vi "RT_MATH_IIR_Filt.vi"(4 "Data In":sgl, 5 "Filter Response (rad/s)":sgl, 6 "Iteration Time Delta(s)":sgl, 7 "Last Data Out":sgl) -> (2 "RC":sgl, 3 "Data Out":sgl)   [LabVIEW 2024]
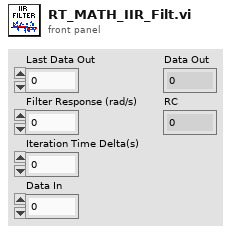
[diagram p1: front panel]
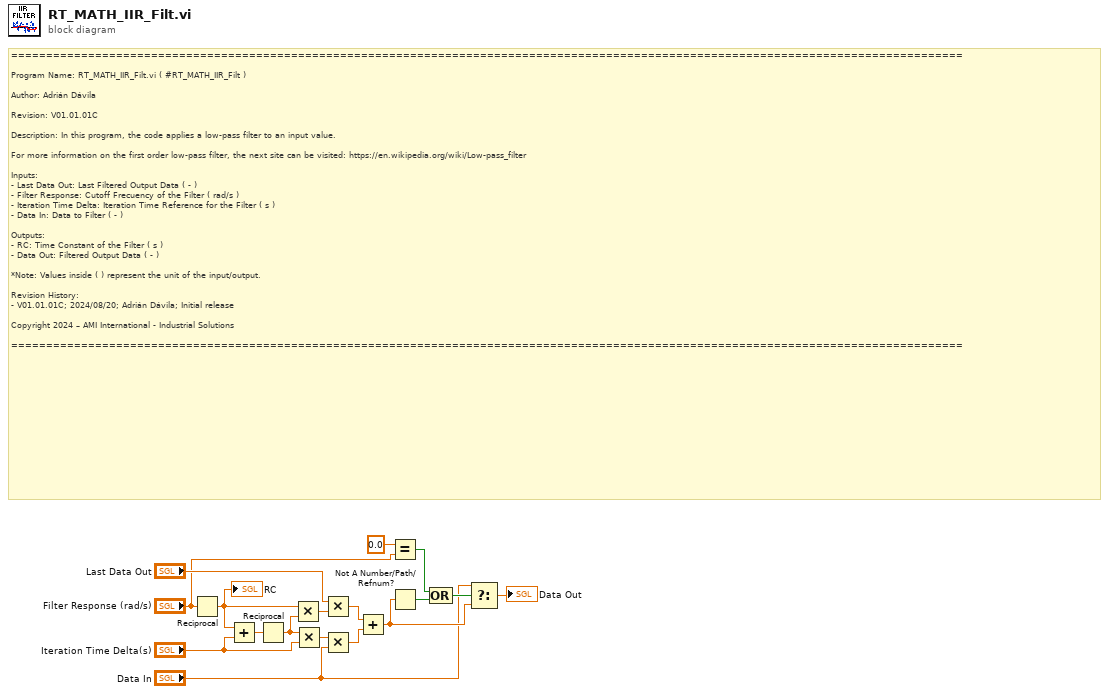
[diagram p0: block diagram]
diagram:
  # "========================================================================================================================================\n\nProgram Name: RT_MATH_IIR_Filt.vi ( #RT_MATH_IIR_Filt )\n\nAuthor: Adrián Dávila\n\nRevision: V01.01.01C\n\nDescription: In this program, the code applies a low-pass filter to an input value.\n\nFor more information on the first order low-pass filter, the next site can be visited: https://en.wikipedia.org/wiki/Low-pass_filter\n\nInputs:\n- Last Data Out: Last Filtered Output Data ( - )\n- Filter Response: Cutoff Frecuency of the Filter ( rad/s ) \n- Iteration Time Delta: Iteration Time Reference for the Filter ( s )\n- Data In: Data to Filter ( - )\n\nOutputs:\n- RC: Time Constant of the Filter ( s )\n- Data Out: Filtered Output Data ( - )\n\n*Note: Values inside ( ) represent the unit of the input/output.\n \nRevision History:\n- V01.01.01C; 2024/08/20; Adrián Dávila; Initial release\n\nCopyright 2024 – AMI International - Industrial Solutions\n\n========================================================================================================================================"
  n1 = Reciprocal(x="Filter Response (rad/s)") -> (1/x=w10:sgl)
  "RC" <- w10
  n2 = Add(x=w10, y="Iteration Time Delta(s)") -> (x+y=w9:sgl)
  n3 = Reciprocal(x=w9) -> (1/x=w8:sgl)
  n4 = Multiply(x=w10, y=w8) -> (x*y=w15:sgl)
  n5 = Multiply(x=w8, y="Iteration Time Delta(s)") -> (x*y=w17:sgl)
  n6 = Multiply(x="Last Data Out", y=w15) -> (x*y=w14:sgl)
  n7 = Multiply(x=w17, y="Data In") -> (x*y=w16:sgl)
  n8 = Add(x=w14, y=w16) -> (x+y=w12:sgl)
  n9 = Equal?(x=sgl 0.0 ("t"), y="Filter Response (rad/s)") -> (x = y?=w3:bool)
  n10 = Not A Number/Path/Refnum?(number/path/refnum=w12) -> (NaN/Path/Refnum?=w6:bool)
  n11 = Compound Arithmetic op=OR(w3, w6) -> (w5:bool)
  n12 = Select(t="Data In", s=w5, f=w12) -> (s? t:f=→"Data Out":sgl)
